vi "DIO_Test.vi"   [LabVIEW 2018]
uses:
  Ctl_IOWriteCommand.ctl
types:
  T1 = typedef "Ctl_IOWriteCommand.ctl" = enum16{"Init", "Set", "ALL_OFF", "Check", "Close"}
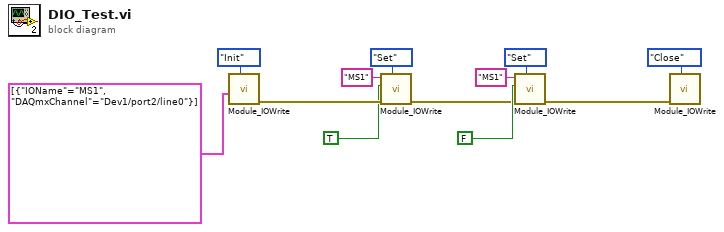
[diagram p0: block diagram]
diagram:
  n1 = call "Module_IOWrite.vi"("IOWrite_Cmd"=Ctl_IOWriteCommand."Init", "IOName-LineName"=cluster{"IOName":string, "DAQmxChannel":tag}[] [{"IOName"="MS1", "DAQmxChannel"="Dev1/port2/line0"}]) -> ("error out"=w10:errorcluster)  [unwired: 7 in, 2 out]
  n2 = call "Module_IOWrite.vi"("IOWrite_Cmd"=Ctl_IOWriteCommand."Set", "error in (no error)"=w10, "ON/OFF"=TRUE, "IOName"="MS1") -> ("error out"=w4:errorcluster)  [unwired: 5 in, 2 out]
  n3 = call "Module_IOWrite.vi"("IOWrite_Cmd"=Ctl_IOWriteCommand."Set", "error in (no error)"=w4, "ON/OFF"=FALSE, "IOName"="MS1") -> ("error out"=w2:errorcluster)  [unwired: 5 in, 2 out]
  n4 = call "Module_IOWrite.vi"("IOWrite_Cmd"=Ctl_IOWriteCommand."Close", "error in (no error)"=w2) -> ()  [unwired: 7 in, 3 out]
